vi "TestSingleTransducer.vi"(6 "Full Range":dbl=300.0, 9 "Reference":dbl, 10 "Analog In":dbl) -> (2 "Pressure":dbl)   [LabVIEW 2019]
panel:
  out "Ref":dbl
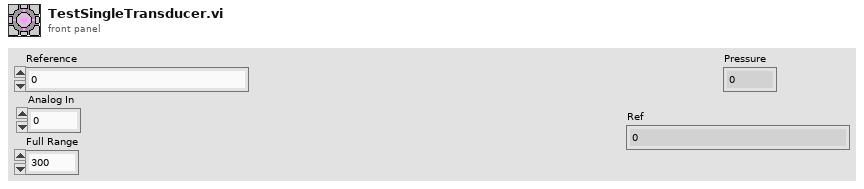
[diagram p1: front panel]
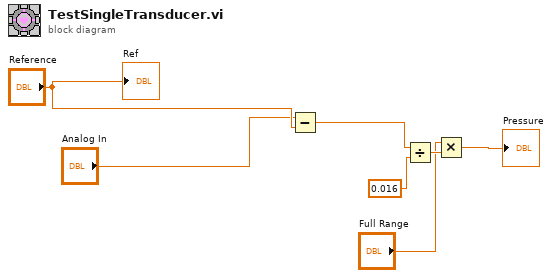
[diagram p0: block diagram]
diagram:
  n1 = Subtract(x="Analog In", y="Reference") -> (x-y=w5:dbl)
  n2 = Divide(x=w5, y=0.016) -> (x/y=w6:dbl)
  n3 = Multiply(x="Full Range", y=w6) -> (x*y=→"Pressure":dbl)
  "Ref" <- "Reference"
